vi "Send Error Criticality.vi"(6 "error in (no error)":errorcluster, 8 "Crit. Level":u8, 9 "Tamer in":refnum<class "Tamer.lvclass">) -> (0 "error out":errorcluster, 3 "Tamer out":refnum<class "Tamer.lvclass">)   [LabVIEW 2020, in "TALOS.lvlib" / "Tamer.lvlib" / "Tamer.lvclass"]
uses:
  Tamer.lvclass
  C:/LabVIEW Code/TALOS/talos/Father of all uServices/Father of all uServices/Father of all uServices.lvclass
  Tamer.lvclass/Tamer.ctl
  Guardian/Guardian Messages/Message to uService Msg/Message to uService Msg.lvclass/Message to uService Msg.ctl
  Ancestor/Ancestor/Ancestor.lvclass/Ancestor.ctl
  Guardian/Guardian Messages/Message to uService Msg/Send Message to uService.vi
  Support VIs/Substitute Error.vi
  Support VIs/Generate Error.vi
  FGV/Error Memory/Get Error Description.vi
  Support VIs/Get PC name.vi
  Ancestor/Ancestor/Read ID.vi
  Support VIs/Get Class Name.vi
  <vilib>/Utility/error.llb/Clear Errors.vi
  FGV/Error Memory/Error Memory Core.vi
  <vilib>/AdvancedString/Delimited String to 1D String Array.vi
  Support VIs/Circus Root Path.vi
  FGV/Error Memory/Error Crt Lvl checker.vi
  FGV/Error Memory/Error Memory Core.vi/40c8088d-b597-4017-91af-faa98e00292e.vi
  FGV/Error Memory/Error Memory Core.vi/d4a3ab98-063c-4e44-b43d-fbdcfe6c2be2.vi
  Father of all uServices/Father of all uServices/Father of all uServices.lvclass
  C:/LabVIEW Code/TALOS/builds/Actor Framework PPL/Actor Framework.lvlibp/1abvi3w/vi.lib/ActorFramework/Actor/Actor.lvclass
  Is status ongoing - enum.vi
  builds/Actor Framework PPL/Actor Framework.lvlibp/1abvi3w/vi.lib/ActorFramework/Actor/Read Caller Enqueuer.vi
  builds/Actor Framework PPL/Actor Framework.lvlibp/1abvi3w/vi.lib/ActorFramework/Message Enqueuer/Enqueue.vi
  Support VIs/Global Memory.vi
  <vilib>/Utility/LVClass/Get LV Class Name.vi
  Support VIs/Is in Packed Library.vi
  Support VIs/TALOS Root path.vi
  Support VIs/Read CSV worksheet.vi
  Support VIs/Global Constants.vi
  <vilib>/Utility/error.llb/General Error Handler.vi
  Support VIs/Error Log.vi
  Guardian/Guardian Messages/Message to uService Msg/Message to uService Msg.lvclass
  Ancestor/Ancestor/Ancestor.lvclass
  <vilib>/Comparison/Equal/Equal Functor/Equal Functor.lvclass
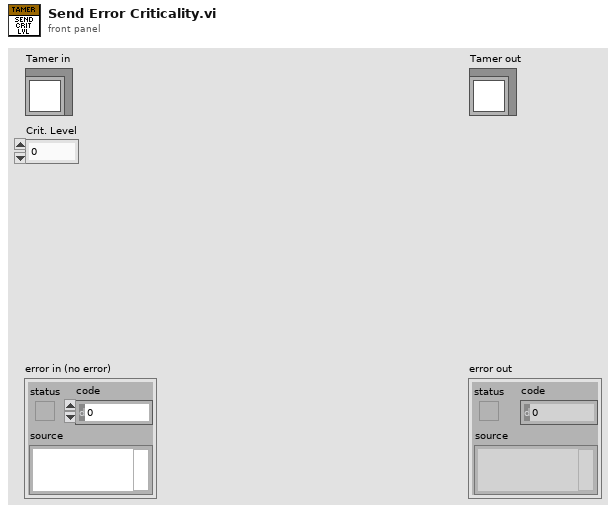
[diagram p1: front panel]
types:
  T1 = typedef "TALOS.lvlib/Run Utilities.lvlib/Monkey Status.ctl" = enum16{"Init", "Paused", "Ongoing", "Stopped", "Finished (no errors)", "Finished (with errors)"}
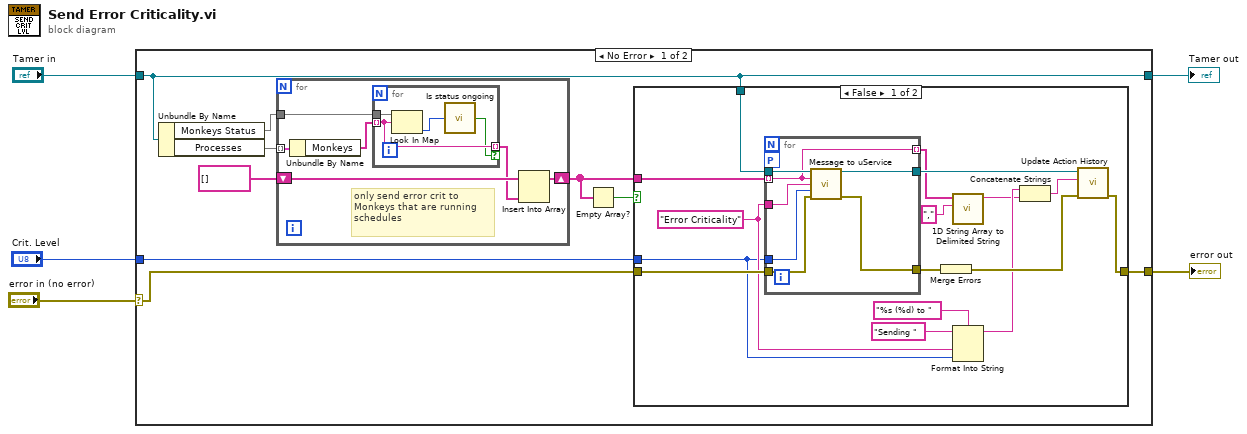
[diagram p0: block diagram]
diagram:
  n1 = case shown="No Error" "error in (no error)" {
    selector: "error in (no error)" -> [w12 w50]
    tunnel: [w14 w50] -> w4
    tunnel: [w11 w49] -> w2
    tunnel: "Tamer in" -> [w11 w49]
    tunnel: "Crit. Level" -> [w9 _]
    frame No Error {
      n2 = Unbundle By Name(w11) -> ("Monkeys Status"=w8:map{string, T1}, "Processes"=w13:map{string, string[]})
      n3 = for {
        tunnel: w13 -> [w44] mode=indexing
        shift-right: [w42] -> w7
        shift-left: string[] [] ("array") -> [w43]
        tunnel: w8 -> [w41]
        # "only send error crit to Monkeys that are running schedules"
        n4 = Unbundle By Name(w44) -> ("Monkeys"=w40:string[])
        n5 = for {
          tunnel: w41 -> [w48]
          tunnel: w40 -> [w46] mode=indexing
          tunnel: [w46] -> w39 mode=indexing if=w45
          n6 = Look In Map(map=w48, key=w46) -> (value=w47:T1)  [unwired: 1 in, 1 out]
          n7 = call-poly "Is status ongoing.vi"("Monkey Status"=w47) -> ("Monkey Running?"=w45:bool)
        }
        n8 = Insert Into Array(array=w43, new element=w39) -> (w42:string[])  [unwired: 1 in]
      }
      n9 = Empty Array?(array=w7) -> (empty?=w6:bool)
      n10 = case shown="False" w6 {
        tunnel: [w29 w38] -> w14
        tunnel: w12 -> [w28 w38]
        tunnel: w7 -> [w27 _]
        tunnel: w11 -> [w26 _]
        tunnel: w9 -> [w20 _]
        frame False {
          w21 = "Error Criticality" ("Message")
          n11 = for {
            tunnel: w21 -> [w34]
            tunnel: w20 -> [w37]
            tunnel: w27 -> [w32] mode=indexing
            tunnel: [w32] -> w18 mode=indexing
            workers-P: _ -> [_]
            tunnel: w28 -> [w36]
            tunnel: [w31] -> w15
            tunnel: w26 -> [w35]
            tunnel: [w33] -> w25
            n12 = call "Message to uService.vi"("Father of all uServices in"=w35, "uService ID"=w32, "Message"=w34, "Data"=w37, "error in (no error)"=w36) -> ("Father of all uServices out"=w33:refnum<class "Tamer.lvclass">, "error out"=w31:errorcluster)  [unwired: 9 in]
          }
          n13 = Merge Errors(w15) -> (w30:errorcluster)
          n14 = call <vilib>:"1D String Array to Delimited String.vi"("delimiter"="," ("Separator"), "string array"=w18) -> ("delimited string"=w16:string)  [unwired: 9 in]
          n15 = Format Into String(format string="%s (%d) to ", initial string="Sending ", w21, w20) -> (resulting string=w19:string)  [unwired: 1 in, 1 out]
          n16 = Concatenate Strings(w19, w16) -> (w24:string)
          n17 = call-dynamic "Update Action History.vi"("error in (no error)"=w30, "Action"=w24, "Tamer in"=w25) -> ("error out"=w29:errorcluster)  [unwired: 7 in, 1 out]
        }
        frame True {
          # "No monkeys running, then we don't have to send the crit level"
        }
      }
    }
    frame Error {
    }
  }
  "error out" <- w4
  "Tamer out" <- w2
